vi "例3.6  滑动杆(简易计算器)3.vi"() -> ()   [LabVIEW 2012]
panel:
  in  "滑动杆":i8(slide) scale=0.0..2.0
  out "Result":dbl
  in  "B":dbl
  in  "A":dbl
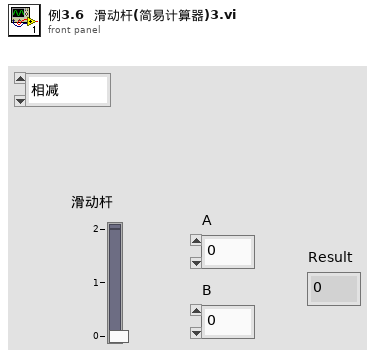
[diagram p1: front panel]
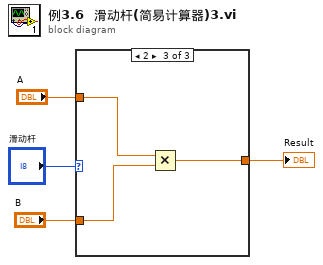
[diagram p0: block diagram]
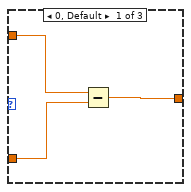
[diagram p2: hidden frame]
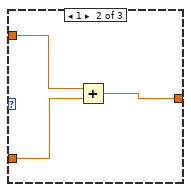
[diagram p3: hidden frame]
diagram:
  n1 = case shown="2" "滑动杆" {
    tunnel: "A" -> [w7 w10 w13]
    tunnel: "B" -> [w6 w9 w12]
    tunnel: [w5 w8 w11] -> w2
    frame 0, Default {
      n2 = Subtract(x=w7, y=w6) -> (x-y=w5:dbl)
    }
    frame 1 {
      n3 = Add(x=w10, y=w9) -> (x+y=w8:dbl)
    }
    frame 2 {
      n4 = Multiply(x=w13, y=w12) -> (x*y=w11:dbl)
    }
  }
  "Result" <- w2
